vi "FGA Get Client Net Location by Source ID.vi"(3 "ID":u32) -> (0 "Record Exists?":bool, 1 "Network Location":T1)   [LabVIEW 2011]
uses:
  UDP Lib/UDP Network Location.ctl
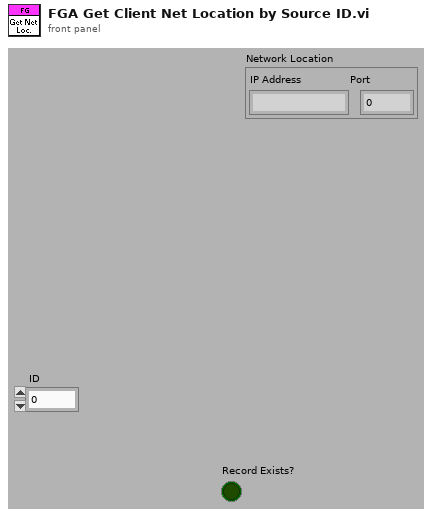
[diagram p1: front panel]
types:
  T1 = typedef "UDP Network Location.ctl" = cluster{"IP Address":string, "Port":u16}
  T2 = typedef "Source ID Network Location Pair.ctl" = cluster{"ID":u32, "Network Location":T1}
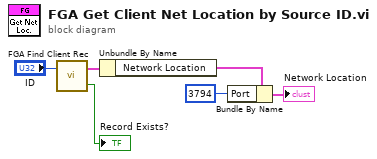
[diagram p0: block diagram]
diagram:
  n1 = call "FGA Find Client Rec.vi"("Source ID"="ID") -> ("Record Exists?"=→"Record Exists?":bool, "Record out"=w4:T2)  [unwired: 1 in]
  n2 = Unbundle By Name(w4) -> ("Network Location"=w3:T1)
  n3 = Bundle By Name(cluster=w3, "Port"=u16 3794) -> (→"Network Location":T1)
